vi "AddCharacter.vi"(8 "error in (no error)":errorcluster, 10 "Character":refnum<class "Character.lvclass">, 11 "reference in":refnum<class "Row.lvclass">) -> (0 "error out":errorcluster, 3 "reference in":refnum<class "Row.lvclass">)   [LabVIEW 2012, in "Row.lvclass"]
uses:
  Row.lvclass
  Character_class/Character.lvclass
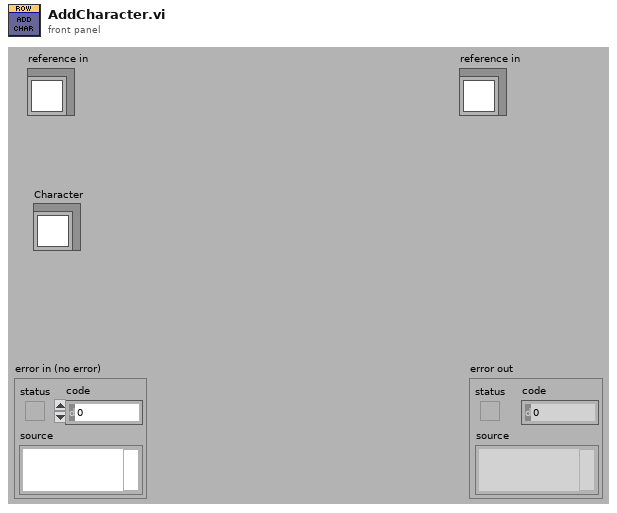
[diagram p1: front panel]
types:
  T1 = typedef "Row.lvclass/ObjectAttributes.ctl" = cluster{"Characters":refnum<class "Character.lvclass">[], "StartPoint":T2, "CharacterSpacing":i32}
  T2 = typedef "Glyph.lvclass/Position.ctl" = cluster{"X":i32, "Y":i32}
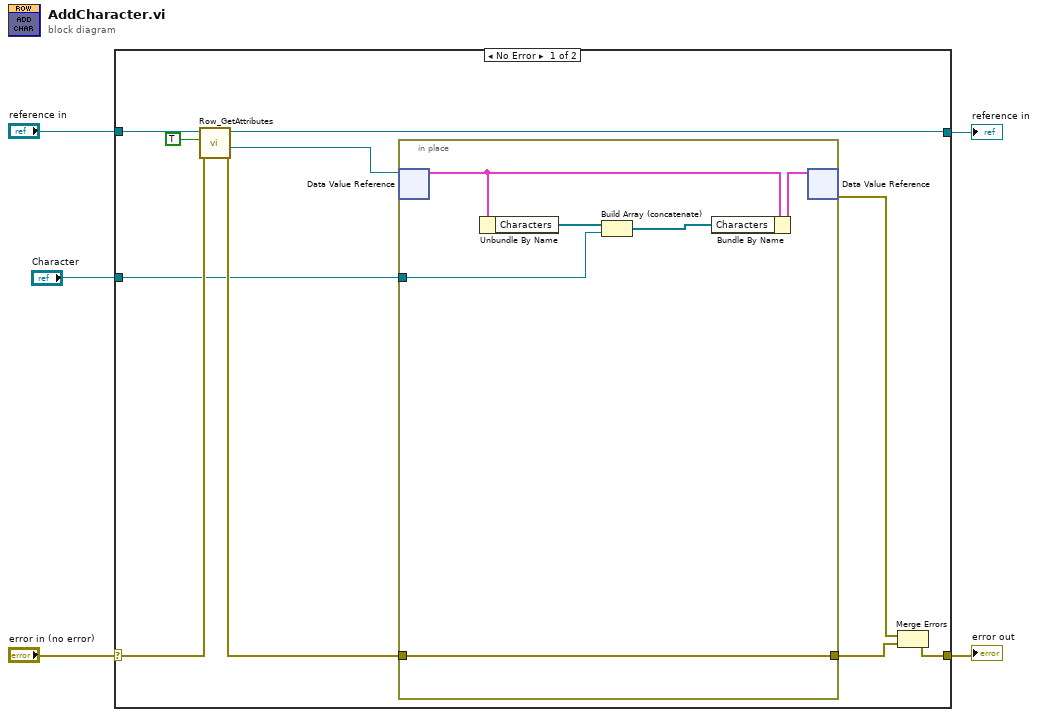
[diagram p0: block diagram]
diagram:
  n1 = case shown="No Error" "error in (no error)" {
    selector: "error in (no error)" -> [w10 w23]
    tunnel: [w14 w23] -> w4
    tunnel: [w12 w22] -> w2
    tunnel: "reference in" -> [w13 w22]
    tunnel: "Character" -> [w6 _]
    frame No Error {
      n2 = call "Row_GetAttributes.vi"("error in (no error)"=w10, "OnlyGetDvrReference(False)"=TRUE, "reference in"=w13) -> ("error out"=w8:errorcluster, "DataRef"=w11:refnum<data-value>, "reference out"=w12:refnum<class "Row.lvclass">)  [unwired: 5 in, 1 out]
      n3 = in-place {
        in-place-border: w8 -> [w20]
        in-place-border: [w20] -> w7
        in-place-border: w6 -> [w16]
        n4 = in-place-dvr #1(w11) -> (w19:T1)  [unwired: 1 out]
        n5 = Unbundle By Name(w19) -> ("Characters"=w18:refnum<class "Character.lvclass">[])
        n6 = Build Array (concatenate)(w18, w16) -> (w17:refnum<class "Character.lvclass">[])
        n7 = Bundle By Name(cluster=w19, "Characters"=w17) -> (w21:T1)
        n8 = in-place-dvr #1(w21) -> (w15:errorcluster)  [unwired: 1 out]
      }
      n9 = Merge Errors(w15, w7) -> (w14:errorcluster)
    }
    frame Error {
    }
  }
  "error out" <- w4
  "reference in" <- w2
